vi "EmergencyStringGLOBAL (1).vi"() -> ()   [LabVIEW 2017]
panel:
  in  "EmergencySource":string
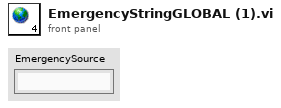
[diagram p1: front panel]
diagram:
